vi "Pockels Cal-Find wavelengths in cal file.vi"(11 "Loaded cal file":string[][](array[string])) -> (2 "Pockels cal'd wavelengths":dbl[](array[numeric]), 3 "Indices of Elements":i32[](array[numeric]))   [LabVIEW 2013]
uses:
  Program Files (x86)/National Instruments/LabVIEW 2013/user.lib/_OpenG.lib/array/array.llb/Search 1D Array (String)__ogtk.vi
  Globals/gl_Calibration globals.vi
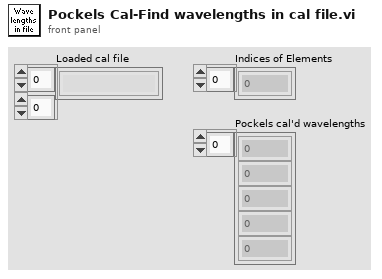
[diagram p1: front panel]
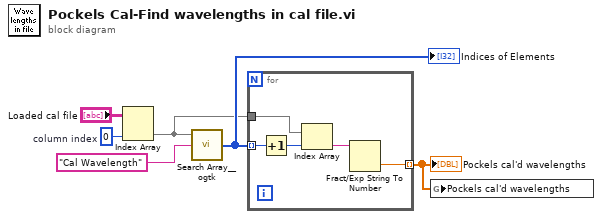
[diagram p0: block diagram]
diagram:
  w2 = 0  # column index
  n1 = Index Array(array="Loaded cal file", index (col)=w2) -> (element=w5:string[])  [unwired: 1 in]
  n2 = call-poly "Search Array__ogtk.vi"("Array"=w5, "Element Data"="Cal Wavelength" ("element")) -> ("Indices of Elements"=w6:i32[])  [unwired: 7 in]
  "Indices of Elements" <- w6
  n3 = for {
    tunnel: w6 -> [w9] mode=indexing
    tunnel: w5 -> [w8]
    tunnel: [w7] -> w1 mode=indexing
    n4 = Increment(x=w9) -> (x+1=w11:i32)
    n5 = Index Array(array=w8, index=w11) -> (element=w10:string)
    n6 = Fract/Exp String To Number(string=w10) -> (number=w7:dbl)  [unwired: 3 in, 1 out]
  }
  "Pockels cal'd wavelengths" <- w1
  n7 = global write "gl_Calibration globals.vi" "Pockels cal'd wavelengths"(w1) -> ()
